vi "get_table.vi"(8 "error in (no error)":errorcluster, 10 "table_name":string, 11 "Doc in":refnum<class "Doc.lvclass">) -> (0 "error out":errorcluster, 1 "Table":refnum<class "Table.lvclass">, 3 "Doc out":refnum<class "Doc.lvclass">)   [LabVIEW 2020, in "toml_edit.lvlib" / "Doc.lvclass"]
uses:
  Doc.lvclass
  Table/Table.lvclass
  Doc.lvclass/Doc.ctl
  dragon_toml_64.dll
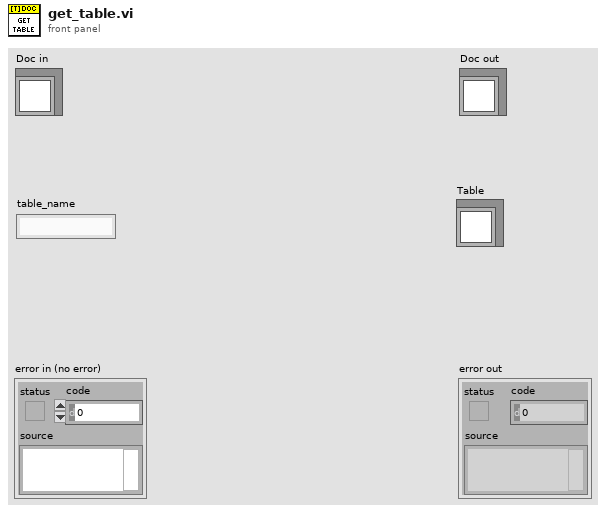
[diagram p1: front panel]
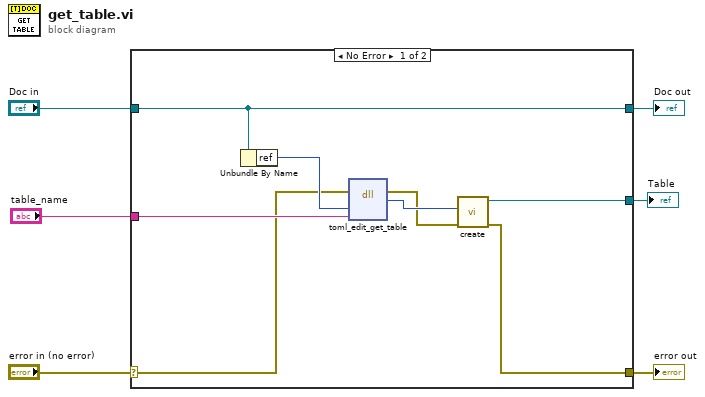
[diagram p0: block diagram]
diagram:
  n1 = case shown="No Error" "error in (no error)" {
    selector: "error in (no error)" -> [w11 w16]
    tunnel: [w7 w16] -> w5
    tunnel: [w13 w15] -> w3
    tunnel: "Doc in" -> [w13 w15]
    tunnel: "table_name" -> [w12 _]
    tunnel: [w8 _] -> w1
    frame No Error {
      n2 = Unbundle By Name(w13) -> ("ref"=w14:u64)
      n3 = dll-call lib="C:/Projects/toml-edit-labview/lv_src/dragon_toml_*.dll" fn="toml_edit_get_table"(error in=w11, "doc_ref"=w14, "table_name"=w12) -> (error out=w9:errorcluster, "table_ptr"=w10:u64)  [unwired: 4 in, 1 out]
      n4 = call "create.vi"("error in (no error)"=w9, "ref"=w10) -> ("error out"=w7:errorcluster, "Table out"=w8:refnum<class "Table.lvclass">)  [unwired: 8 in]
    }
    frame Error {
    }
  }
  "error out" <- w5
  "Doc out" <- w3
  "Table" <- w1
